vi "ArmPressureCalcMethodSettings.vi"(11 "notifier":refnum<notifier>) -> ()   [LabVIEW 2013, in "main.lvlib"]
uses:
  main.lvlib
  Controls/Enum Variables.ctl
  Controls/Enum Save Action Events.ctl
panel:
  in  "armPressCalcDescriptions":string[](array[string])=["Beregner det gennemsnitlige tryk ud fra alle de indtastede værdier for hver kolonne. ", "Beregner det gennemsnitlige tryk for hver kolonne. Som indeks bruges det højeste gennemsnit af højre eller venstre. ", "Forkaster tryk som er mere end én standard afvigelse under det gennemsnitlige tryk. Beregner gennemsnitligt tryk for de resterende. "]
  out "armPressureDescriptionString":string="Beregner det gennemsnitlige tryk ud fra alle de indtastede værdier for hver kolonne. " caption="Description"
  in  "Calculation Type":T1(ring) caption="Vælg metode til udregning af amtryk"
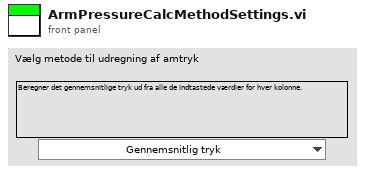
[diagram p1: front panel]
types:
  T1 = enum16{"Gennemsnitlig tryk", "Maksimalt tryk", "Dynamisk middel"}
  T2 = typedef "main.lvlib/Enum Variables.ctl" = enum16{"SetAcqFilter", "GetAcqFilter", "Set Filter", "Get Filter", "Set Height", "Get Height", "Set Recorded Height", "Get Recorded Height", "Set Blue Pressure", "Get Blue Pressure", "Set Red Pressure", "Get Red Pressure", "Init", "Reset Pressure", "Set Red Cursors", "Get Red Cursors", "Set Blue Cursors", "Get Blue Cursors", "Set Language", "Get Language", "Set Active Graphs", "Get ActiveGraphs", "Set Method", "Get Method", "Set Encryption", "Get Encryption", "Set ExcelVersion", "Get ExcelVersion", "Set DICOM Avail", "Get DICOM Avail", "Set DICOM Encode", "Get DICOM Encode", "Set JournalExport", "Get JournalExport", "Set Sequence", "Get Sequence", "Set DAQ Connected", "Get DAQ Connected", "Set Current Graph", "Get Current Graph", "Set General Settings", "Get Hyphenation", "Set Arm Calc Method", "Get Arm Calc Method", "Set Dicom Tags", "Get Dicom Tags", "Set BT Serial", "Get BT Serial", "Set BT Accepted Serials", "Get BT Accepted Serials", "Get BT License", "Set BT License"}
  T3 = typedef "main.lvlib/Enum Save Action Events.ctl" = enum16{"LoadReportPath", "SaveReportPath", "Load Graph Path", "Save Graph Path", "LoadDataPath", "SaveDataPath", "Load Template Path", "Save Template Path", "Load PressureFactor", "Save PressureFactor", "Init", "Load Listbox", "Save Listbox", "LoadHospInfo", "SaveHospInfo", "Load DICOM Activation", "Save DICOM Activation", "LoadDICOMInfoWL", "SaveDICOMInfoWL", "LoadDICOMInfoPACS", "SaveDICOMInfoPACS", "Load ArmCalcMethod", "Save ArmCalcMethod", "LoadItemTags", "SaveItemTags", "LoadDICOMEncoding", "SaveDICOMEncoding", "LoadJournalType", "SaveJournalType", "LoadAcqFilterType", "SaveAcqFilterType", "Load Sequence", "Save Sequence", "Load Acquisition Mode", "Save Acquisition Mode", "Load General Settings", "Save General Settings", "Load Language", "Save Language", "Load Dicom Tags", "Save Dicom Tags", "Load BT Serial", "Save BT Serial", "Load BT License", "Save BT License"}
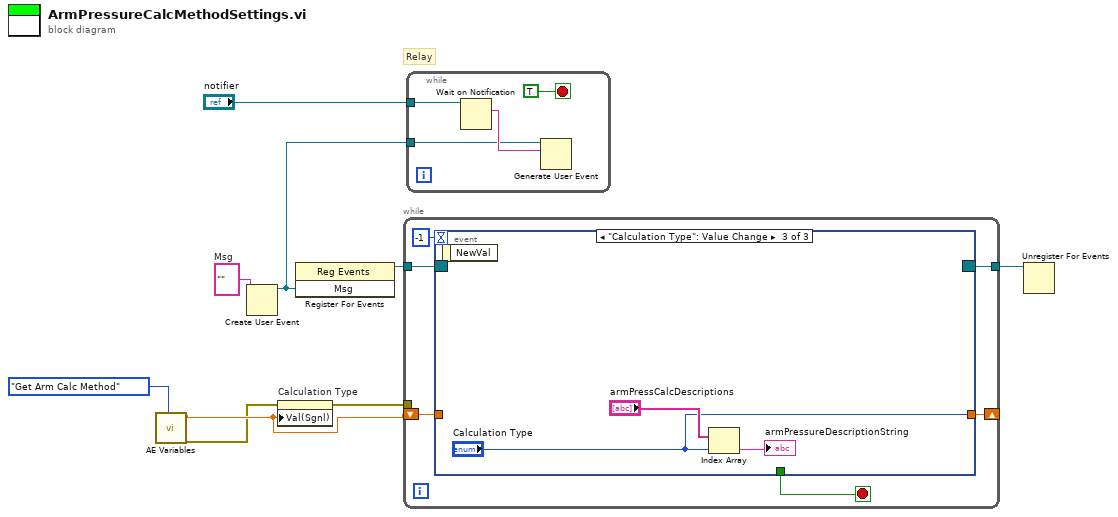
[diagram p0: block diagram]
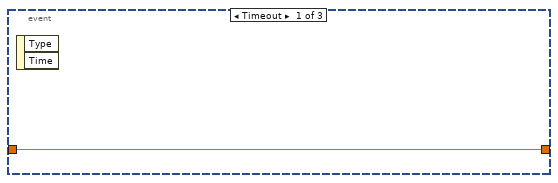
[diagram p2: hidden frame]
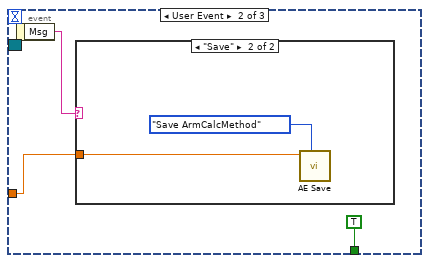
[diagram p3: hidden frame]
diagram:
  w8 = ""  # Msg
  # "Relay"
  n1 = call "AE Variables.vi"("Action"=Enum_Variables."Get Arm Calc Method") -> ("NumericOut"=w2:dbl, "error out"=w1:errorcluster)  [unwired: 11 in, 6 out]
  n2 = Create User Event(user event datatype=w8) -> (user event=w7:refnum<user-event>)  [unwired: 1 in, 1 out]
  n3 = property on="Calculation Type" class="Enum (strict)"(error in=w1, "Val(Sgnl)"=w2) -> (error out=w6:errorcluster)  [unwired: 1 in, 1 out]
  n4 = register-events(w7) -> (reference out=w5:refnum<event-registration>)  [unwired: 2 in, 1 out]
  n5 = while {
    tunnel: w5 -> [w15]
    tunnel: w6 -> [_]
    shift-right: [w12] -> _
    shift-left: w2 -> [w11]
    tunnel: [w10] -> w4
    stop <- w14 stop-if-true
    n6 = event shown="[2] \"Calculation Type\": Value Change" {
      selector: w15 -> [_ _ _]
      dyn-events: [_ _ _] -> w10
      timeout: -1 -> [_ _ _]
      tunnel: [_ TRUE _] -> w14
      tunnel: [w16 _ "Calculation Type"] -> w12
      tunnel: w11 -> [w16 w17 _]
      event Timeout {
        n7 = event-data() -> ()  [unwired: 1 in, 2 out]
      }
      event User Event {
        n8 = event-data() -> ("Msg"=w18:string)  [unwired: 1 in]
        n9 = case shown="\"Save\"" w18 {
          tunnel: w17 -> [_ w21]
          frame "Cancel", Default {
          }
          frame "Save" {
            n10 = call "AE Save.vi"("Variant In"=w21, "Action"=Enum_Save_Action_Events."Save ArmCalcMethod") -> ()  [unwired: 7 in, 2 out]
          }
        }
      }
      event "Calculation Type": Value Change {
        n11 = event-data() -> ()  [unwired: 1 in, 1 out]
        n12 = Index Array(array="armPressCalcDescriptions", index="Calculation Type") -> (element=→"armPressureDescriptionString":string)
      }
    }
  }
  n13 = while {
    tunnel: "notifier" -> [w28]
    tunnel: w7 -> [w25]
    stop <- TRUE stop-if-true
    n14 = Wait on Notification(notifier=w28) -> (notification=w26:string)  [unwired: 3 in, 3 out]
    n15 = Generate User Event(user event=w25, event data cluster=w26) -> ()  [unwired: 2 in, 2 out]
  }
  n16 = Unregister For Events(event registration refnum=w4) -> ()  [unwired: 1 in, 1 out]
